vi "ConfigureWfrm.vi"(8 "error in (no error)":errorcluster, 10 "SampleRate":dbl=1000.0, 11 "MultiBandState in":refnum<class "MultiBandState.lvclass">) -> (0 "error out":errorcluster, 3 "MultiBandState out":refnum<class "MultiBandState.lvclass">)   [LabVIEW 2018, in "Functions.lvlib" / "MultiBandState.lvclass"]
uses:
  MultiBandState.lvclass
  MultiBandState.lvclass/MultiBandState.ctl
  Accessors/Write SampleRate.vi
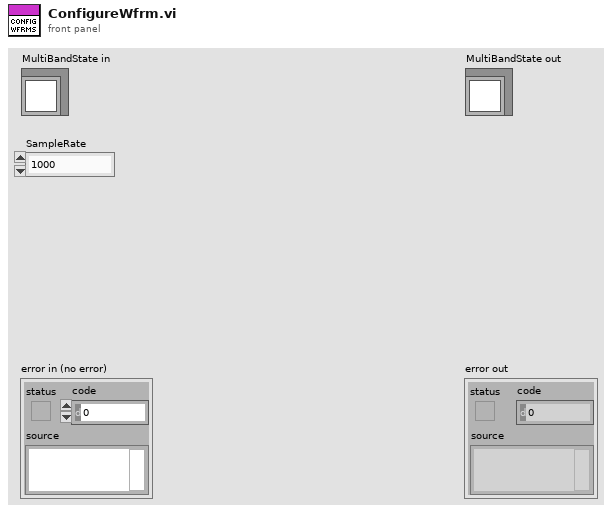
[diagram p1: front panel]
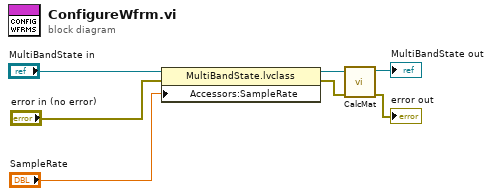
[diagram p0: block diagram]
diagram:
  n1 = property class="MultiBandState.lvclass"(reference="MultiBandState in", error in="error in (no error)", "Accessors:SampleRate"="SampleRate") -> (reference out=w4:refnum<class "MultiBandState.lvclass">, error out=w3:errorcluster)
  n2 = call "CalcMat.vi"("error in (no error)"=w3, "MultiBandState in"=w4) -> ("error out"=→"error out":errorcluster, "MultiBandState out"=→"MultiBandState out":refnum<class "MultiBandState.lvclass">)  [unwired: 8 in]
